vi "State_Machine.vi"() -> ()   [LabVIEW 2022 SP3]
uses:
  SM_States.ctl
  SM_Data.ctl
  <vilib>/numeric/Random Number (Range) DBL.vi
panel:
  out "Info":T1
  in  "Stop":bool
  in  "Run Cleaning":bool
  in  "SM_Data":T1
  in  "SM_States":T2=enum."Init"
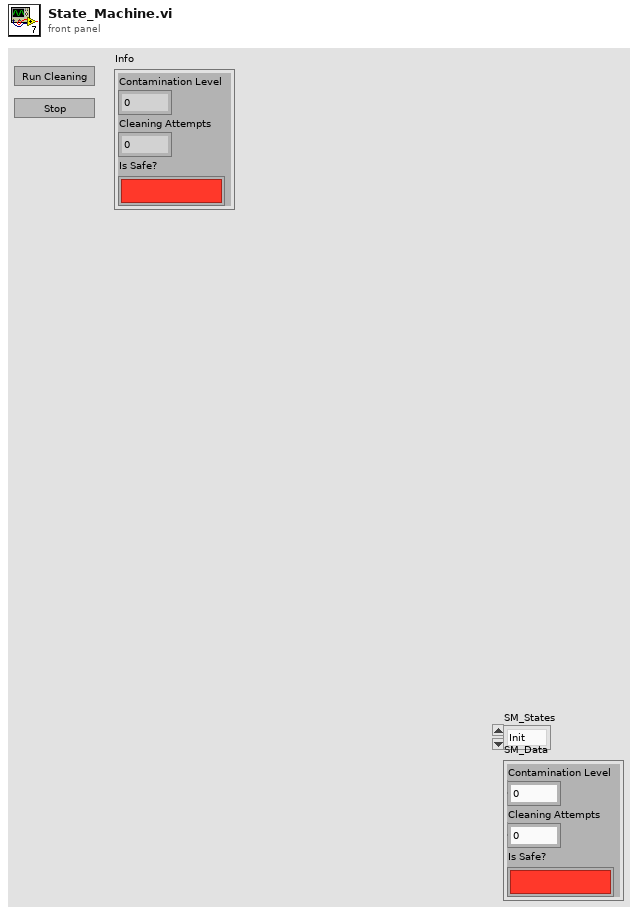
[diagram p1: front panel]
types:
  T1 = typedef "SM_Data.ctl" = cluster{"Contamination Level":dbl, "Cleaning Attempts":dbl, "Is Safe?":bool}
  T2 = typedef "SM_States.ctl" = enum16{"Clean", "Check Contamination", "Stop", "Init", "Idle"}
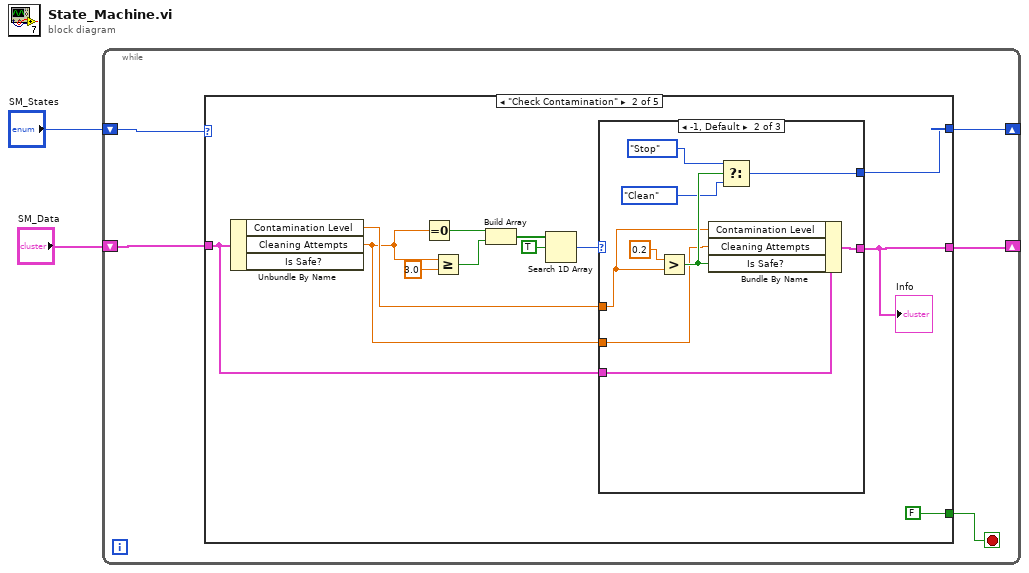
[diagram p0: block diagram]
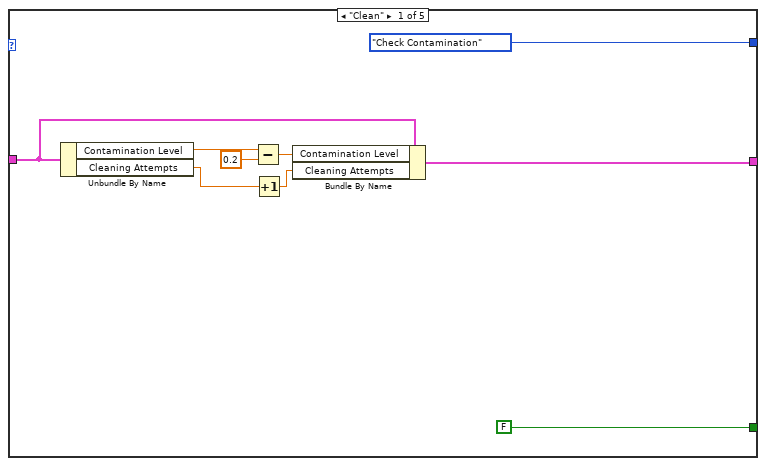
[diagram p2: hidden frame]
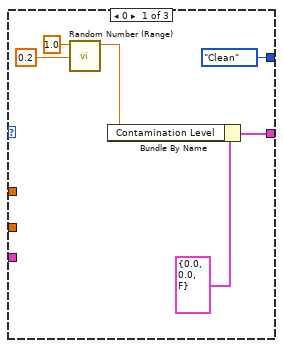
[diagram p3: hidden frame]
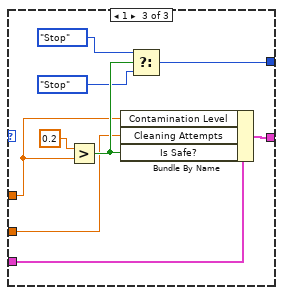
[diagram p4: hidden frame]
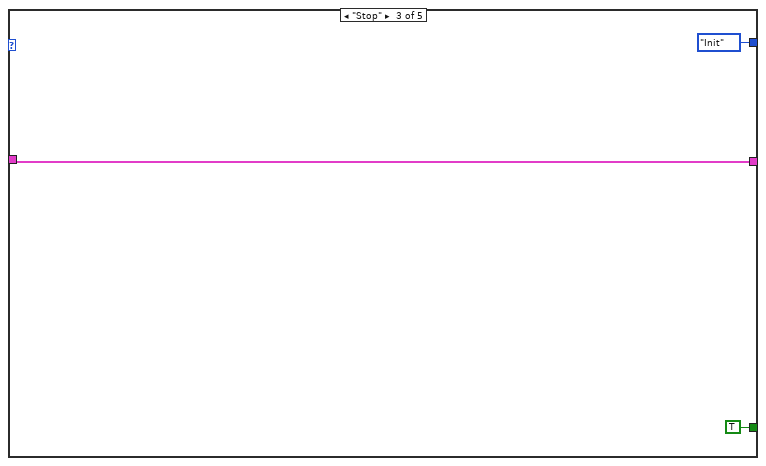
[diagram p5: hidden frame]
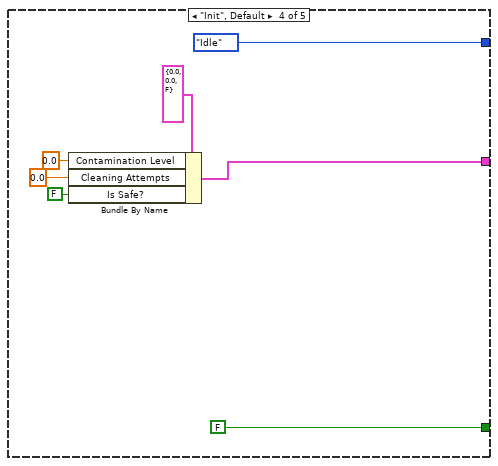
[diagram p6: hidden frame]
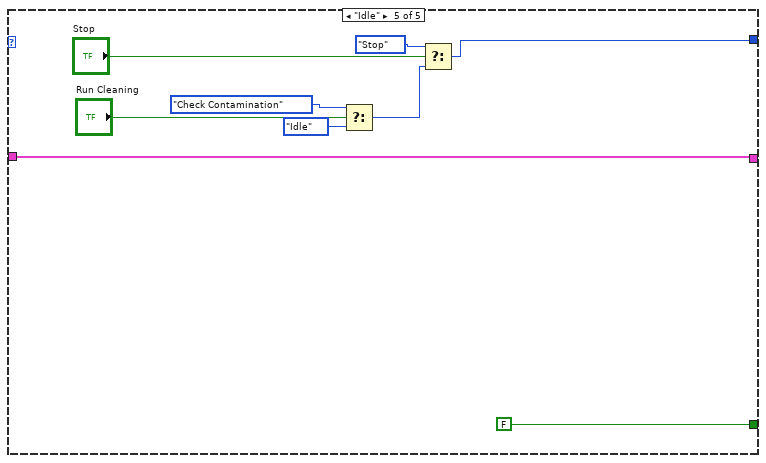
[diagram p7: hidden frame]
diagram:
  n1 = while {
    shift-right: [w5] -> _
    shift-left: "SM_States" -> [w7]
    shift-right: [w6] -> _
    shift-left: "SM_Data" -> [w3]
    stop <- w4 stop-if-true
    n2 = case shown="\"Check Contamination\"" w7 {
      tunnel: [w9 w20 w55 w61 w71] -> w6
      tunnel: [SM_States."Check Contamination" ("f") w22 SM_States."Init" ("f") SM_States."Idle" ("SM_States") w64] -> w5
      tunnel: [FALSE FALSE TRUE FALSE FALSE] -> w4
      tunnel: w3 -> [w12 w21 w55 _ w71]
      frame "Clean" {
        n3 = Unbundle By Name(w12) -> ("Contamination Level"=w15:dbl, "Cleaning Attempts"=w13:dbl)
        n4 = Subtract(x=w15, y=0.2) -> (x-y=w11:dbl)
        n5 = Increment(x=w13) -> (x+1=w10:dbl)
        n6 = Bundle By Name(cluster=w12, "Contamination Level"=w11, "Cleaning Attempts"=w10) -> (w9:T1)
      }
      frame "Check Contamination" {
        n7 = Unbundle By Name(w21) -> ("Contamination Level"=w23:dbl, "Cleaning Attempts"=w17:dbl)  [unwired: 1 out]
        n8 = Equal To 0?(x=w17) -> (x = 0?=w18:bool)
        n9 = Greater Or Equal?(x=w17, y=3.0) -> (x >= y?=w28:bool)
        n10 = Build Array(w18, w28) -> (w27:bool[])
        n11 = Search 1D Array(1D array=w27, element=TRUE) -> (index of element=w24:i32)  [unwired: 1 in]
        n12 = case shown="-1, Default" w24 {
          tunnel: w23 -> [_ w36 w44]
          tunnel: [w30 w37 w46] -> w20
          tunnel: [SM_States."Clean" ("f") w39 w48] -> w22
          tunnel: w21 -> [_ w38 w47]
          tunnel: w17 -> [_ w35 w45]
          frame 0 {
            n13 = call-poly <vilib>:"Random Number (Range).vi"("lower bound (0)"=0.2, "upper bound (100)"=1.0) -> ("number"=w31:dbl)  [unwired: 9 in]
            n14 = Bundle By Name(cluster=T1 {"Contamination Level"=0.0, "Cleaning Attempts"=0.0, "Is Safe?"=FALSE} ("SM_Data"), "Contamination Level"=w31) -> (w30:T1)
          }
          frame -1, Default {
            n15 = Greater?(x=0.2 ("y"), y=w36) -> (0:w42:bool)
            n16 = Bundle By Name(cluster=w38, "Contamination Level"=w36, "Cleaning Attempts"=w35, "Is Safe?"=w42) -> (w37:T1)
            n17 = Select(t=SM_States."Stop" ("f"), s=w42, f=SM_States."Clean") -> (s? t:f=w39:T2)
          }
          frame 1 {
            n18 = Greater?(x=0.2 ("y"), y=w44) -> (0:w51:bool)
            n19 = Bundle By Name(cluster=w47, "Contamination Level"=w44, "Cleaning Attempts"=w45, "Is Safe?"=w51) -> (w46:T1)
            n20 = Select(t=SM_States."Stop" ("f"), s=w51, f=SM_States."Stop") -> (s? t:f=w48:T2)
          }
        }
        "Info" <- w20
      }
      frame "Stop" {
      }
      frame "Init", Default {
        n21 = Bundle By Name(cluster=T1 {"Contamination Level"=0.0, "Cleaning Attempts"=0.0, "Is Safe?"=FALSE} ("SM_Data"), "Contamination Level"=0.0, "Cleaning Attempts"=0.0, "Is Safe?"=FALSE) -> (w61:T1)
      }
      frame "Idle" {
        n22 = Select(t=SM_States."Check Contamination" ("SM_States"), s="Run Cleaning", f=SM_States."Idle") -> (s? t:f=w65:T2)
        n23 = Select(t=SM_States."Stop" ("SM_States"), s="Stop", f=w65) -> (s? t:f=w64:T2)
      }
    }
  }
